vi "pause3.vi"() -> ()   [LabVIEW 2020]
panel:
  in  "pause3":bool
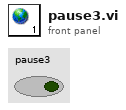
[diagram p1: front panel]
diagram:
